vi "Sum_of_Sines.vi"() -> ()   [LabVIEW 2022 SP3]
panel:
  out "Waveform Graph":dbl[](graph)
  in  "N":i32
  # "Sum of Signs:\nAdjust the value of N to see \nwhat a sum of N sine functions\n would look like."
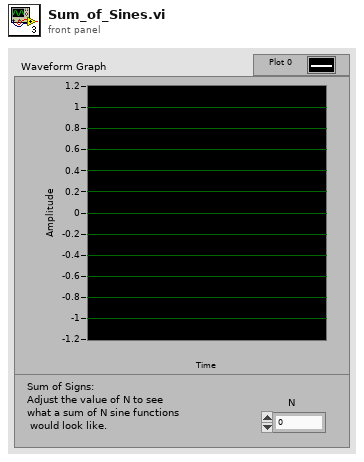
[diagram p1: front panel]
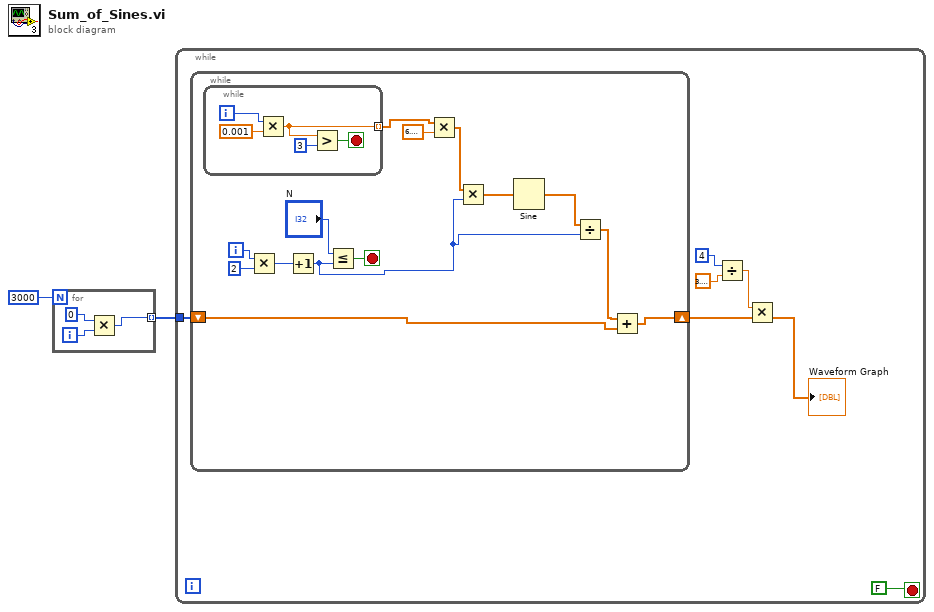
[diagram p0: block diagram]
diagram:
  n1 = for {
    N: 3000 -> [_]
    tunnel: [w3] -> w2 mode=indexing
    i -> [w5]
    n2 = Multiply(x=0, y=w5) -> (x*y=w3:i32)
  }
  n3 = while {
    tunnel: w2 -> [w12]
    stop <- FALSE stop-if-true
    n4 = while {
      shift-right: [w14] -> w11
      shift-left: w12 -> [w13]
      i -> [w26]
      stop <- w22 stop-if-true
      n5 = while {
        tunnel: [w27] -> w20 mode=indexing
        i -> [w31]
        stop <- w28 stop-if-true
        n6 = Multiply(x=w31, y=0.001) -> (x*y=w27:dbl)
        n7 = Greater?(x=w27, y=3) -> (0:w28:bool)
      }
      n8 = Multiply(x=w26, y=2) -> (x*y=w24:i32)
      n9 = Increment(x=w24) -> (x+1=w16:i32)
      n10 = Less Or Equal?(x="N", y=w16) -> (x <= y?=w22:bool)
      n11 = Multiply(x=w20, y=6.283185307179586) -> (x*y=w19:dbl[])
      n12 = Multiply(x=w19, y=w16) -> (x*y=w18:dbl[])
      n13 = Sine(x=w18) -> (sin(x)=w17:dbl[])
      n14 = Divide(x=w17, y=w16) -> (x/y=w15:dbl[])
      n15 = Add(x=w15, y=w13) -> (x+y=w14:dbl[])
    }
    n16 = Divide(x=4, y=3.141592653589793) -> (x/y=w7:dbl)
    n17 = Multiply(x=w7, y=w11) -> (x*y=→"Waveform Graph":dbl[])
  }
